vi "From String.vi"(8 "error in (no error)":errorcluster, 10 "data":string, 11 "OnTheFlyReport Config in":refnum<class "OnTheFlyReport Config.lvclass">) -> (0 "error out":errorcluster, 3 "OnTheFlyReport Config out":refnum<class "OnTheFlyReport Config.lvclass">)   [LabVIEW 2015, in "OnTheFlyReport Config.lvclass"]
uses:
  OnTheFlyReport Config.lvclass
  OnTheFlyReport Config.lvclass/OnTheFlyReport Config.ctl
  Report Formatters/Base Class/Config/Formatter Config.lvclass
  <vilib>/NI/Configuration Framework/serializable configuration/NISE_CEF_serializable configuration.lvclass
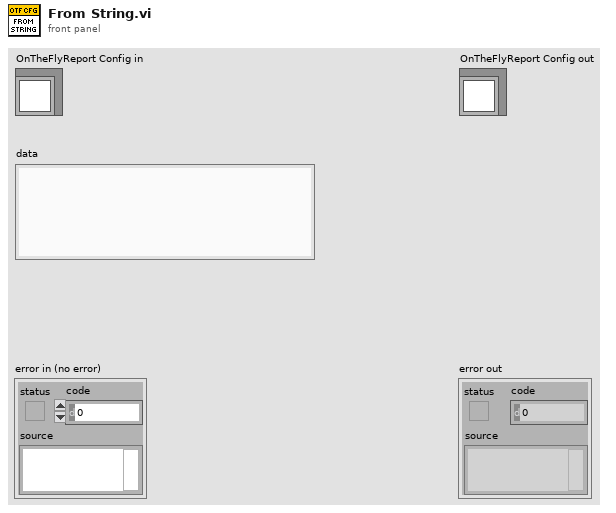
[diagram p1: front panel]
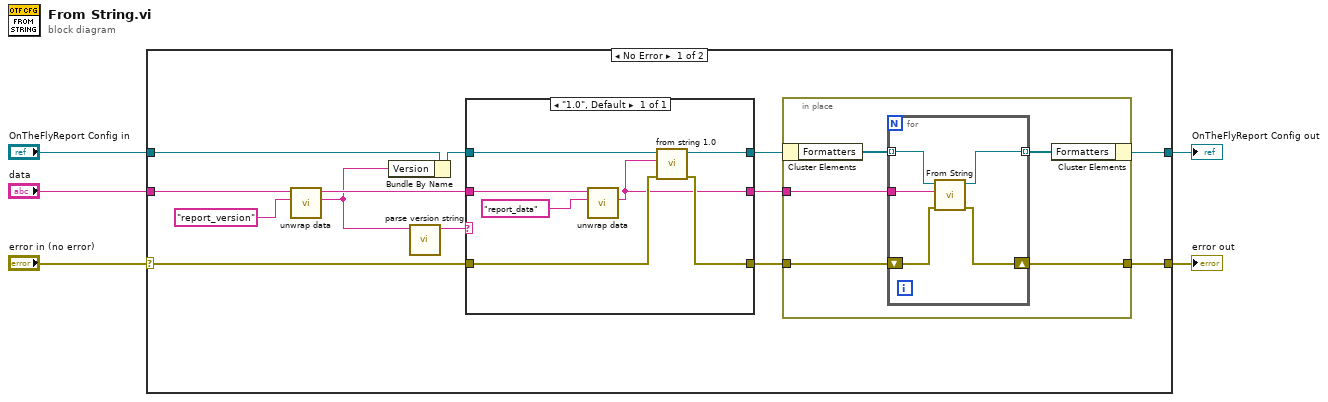
[diagram p0: block diagram]
diagram:
  n1 = case shown="No Error" "error in (no error)" {
    selector: "error in (no error)" -> [w17 w37]
    tunnel: [w12 w37] -> w4
    tunnel: [w14 w36] -> w3
    tunnel: "OnTheFlyReport Config in" -> [w18 w36]
    tunnel: "data" -> [w9 _]
    frame No Error {
      n2 = call <vilib>:"unwrap data.vi"("identifier"="report_version", "data to unwrap"=w9) -> ("unwrapped data"=w6:string, "remaining string"=w10:string)  [unwired: 8 in]
      n3 = Bundle By Name(cluster=w18, "Version"=w6) -> (w7:refnum<class "OnTheFlyReport Config.lvclass">)
      n4 = call <vilib>:"parse version string.vi"("full version"=w6) -> ("major.minor version"=w16:string)  [unwired: 7 in, 3 out]
      n5 = case shown="\"1.0\", Default" w16 {
        tunnel: w10 -> [w35]
        tunnel: w7 -> [w33]
        tunnel: w17 -> [w32]
        tunnel: [w31] -> w13
        tunnel: [w30] -> w15
        tunnel: [w29] -> w11
        frame "1.0", Default {
          n6 = call <vilib>:"unwrap data.vi"("identifier"="report_data", "data to unwrap"=w35) -> ("unwrapped data"=w29:string)  [unwired: 8 in, 1 out]
          n7 = call-dynamic "from string 1.0.vi"("error in (no error)"=w32, "data"=w29, "OnTheFlyReport Config in"=w33) -> ("error out"=w31:errorcluster, "OnTheFlyReport Config out"=w30:refnum<class "OnTheFlyReport Config.lvclass">)  [unwired: 7 in]
        }
      }
      n8 = in-place {
        in-place-border: w13 -> [w22]
        in-place-border: [w21] -> w12
        in-place-border: w11 -> [w19]
        n9 = in-place-cluster #1(w15) -> ("Formatters"=w23:refnum<class "Formatter Config.lvclass">[])
        n10 = for {
          tunnel: w23 -> [w28] mode=indexing
          shift-right: [w25] -> w21
          shift-left: w22 -> [w26]
          tunnel: [w27] -> w20 mode=indexing
          tunnel: w19 -> [w24]
          n11 = call-dynamic "From String.vi"("error in (no error)"=w26, "data"=w24, "Formatter Config in"=w28) -> ("error out"=w25:errorcluster, "Formatter Config out"=w27:refnum<class "Formatter Config.lvclass">)  [unwired: 7 in]
        }
        n12 = in-place-cluster #1("Formatters"=w20) -> (w14:refnum<class "OnTheFlyReport Config.lvclass">)
      }
    }
    frame Error {
    }
  }
  "error out" <- w4
  "OnTheFlyReport Config out" <- w3
